vi "Shooter Elevate.vi"(8 "Elevation Input":enum16{"Down", "Elevating", "Up", "Lowering"}(ring), 9 "Elevation time (s)":dbl, 10 "Lowering time (s)":dbl=1.0, 11 "Elevation Button":bool) -> (0 "Elevation Output":enum16{"Down", "Elevating", "Up", "Lowering"}(ring), 2 "Elevation Solenoid Output":T1)   [LabVIEW 2012]
uses:
  <vilib>/Rock Robotics/WPI/Solenoid/WPI_SolenoidValue.ctl
panel:
  out "State":string
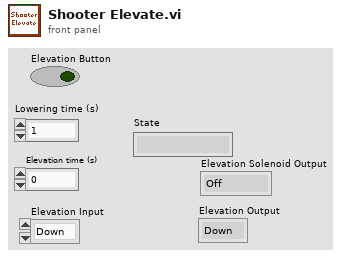
[diagram p1: front panel]
types:
  T1 = typedef "WPI_SolenoidValue.ctl" = enum16{"Off", "On", "Forward", "Reverse"}
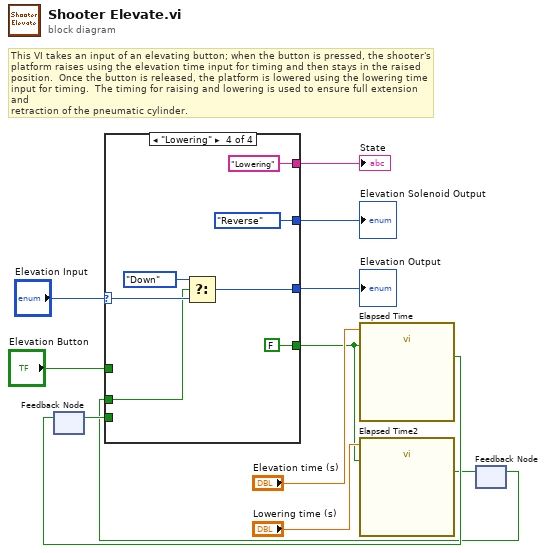
[diagram p0: block diagram]
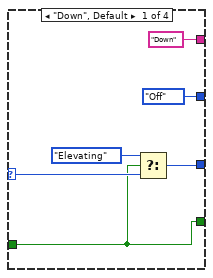
[diagram p2: hidden frame]
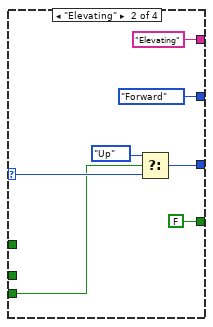
[diagram p3: hidden frame]
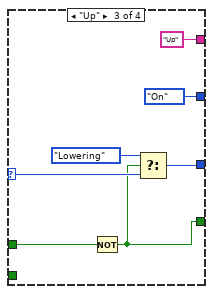
[diagram p4: hidden frame]
diagram:
  # "This VI takes an input of an elevating button; when the button is pressed, the shooter's\nplatform raises using the elevation time input for timing and then stays in the raised position.  Once the button is released, the platform is lowered using the lowering time\ninput for timing.  The timing for raising and lowering is used to ensure full extension and\nretraction of the pneumatic cylinder."
  n1 = feedback #1() -> (w8:bool)  [unwired: 1 in]
  n2 = feedback #2() -> (w4:bool)  [unwired: 1 in]
  n3 = case shown="\"Lowering\"" "Elevation Input" {
    selector: "Elevation Input" -> [w18 w25 w28 w39]
    tunnel: "Elevation Button" -> [w14 _ w30 _]
    tunnel: [w16 w23 w32 w37] -> w12
    tunnel: ["Down" "Elevating" "Up" "Lowering"] -> w11
    tunnel: [w14 FALSE ("Elevate/lower") w27 FALSE ("Elevate/lower")] -> w6
    tunnel: w8 -> [_ w21 _ _]
    tunnel: w4 -> [_ _ _ w34]
    tunnel: [WPI_SolenoidValue."Off" ("Value") WPI_SolenoidValue."Forward" ("Value") WPI_SolenoidValue."On" ("Value") WPI_SolenoidValue."Reverse" ("Value")] -> w2
    frame "Down", Default {
      n4 = Select(t=enum16{"Down", "Elevating", "Up", "Lowering"}."Elevating", s=w14, f=w18) -> (s? t:f=w16:enum16{"Down", "Elevating", "Up", "Lowering"})
    }
    frame "Elevating" {
      n5 = Select(t=enum16{"Down", "Elevating", "Up", "Lowering"}."Up", s=w21, f=w25) -> (s? t:f=w23:enum16{"Down", "Elevating", "Up", "Lowering"})
    }
    frame "Up" {
      n6 = Not(x=w30) -> (.not. x?=w27:bool)
      n7 = Select(t=enum16{"Down", "Elevating", "Up", "Lowering"}."Lowering", s=w27, f=w28) -> (s? t:f=w32:enum16{"Down", "Elevating", "Up", "Lowering"})
    }
    frame "Lowering" {
      n8 = Select(t=enum16{"Down", "Elevating", "Up", "Lowering"}."Down", s=w34, f=w39) -> (s? t:f=w37:enum16{"Down", "Elevating", "Up", "Lowering"})
    }
  }
  "State" <- w11
  "Elevation Output" <- w12
  "Elevation Solenoid Output" <- w2
  n9 = call "Elapsed Time"("Time Target (s)"="Elevation time (s)", "Reset"=w6) -> ("Time has Elapsed"=w9:bool)  [unwired: 10 in, 7 out]
  n10 = feedback-in #1(w9) -> ()
  n11 = call "Elapsed Time2"("Time Target (s)"="Lowering time (s)", "Reset"=w6) -> ("Time has Elapsed"=w5:bool)  [unwired: 10 in, 7 out]
  n12 = feedback-in #2(w5) -> ()
